vi "Response Type.vi"(8 "error in (no error)":errorcluster, 11 "http-client in":refnum<class "http-client.lvclass">) -> (0 "error out":errorcluster, 2 "response type":refnum<class "response.lvclass">, 3 "http-client out":refnum<class "http-client.lvclass">)   [LabVIEW 2020, in "http.lvlib" / "http-client.lvclass"]
uses:
  http-client.lvclass
  response/response.lvclass
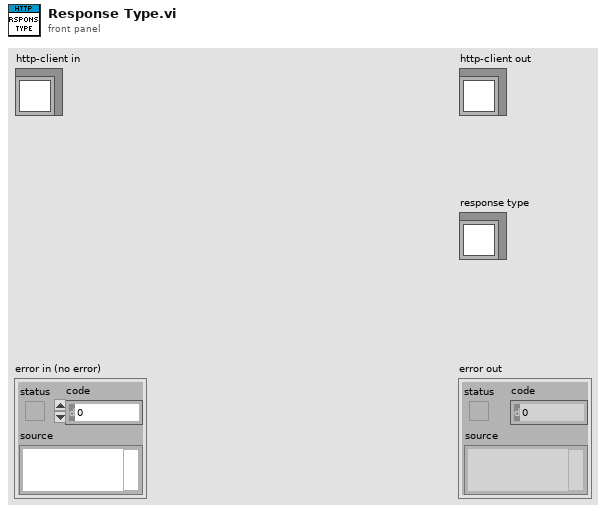
[diagram p1: front panel]
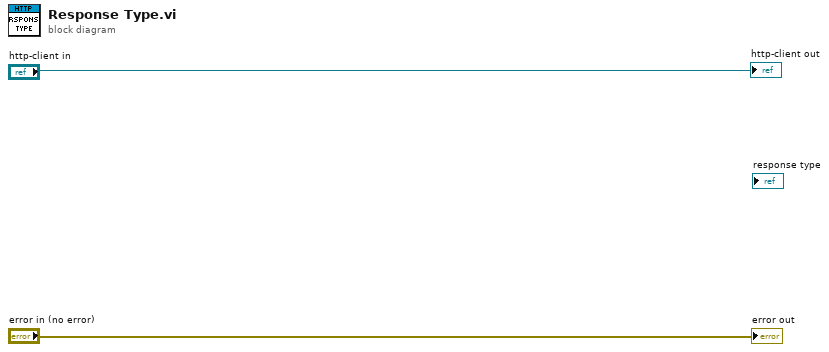
[diagram p0: block diagram]
diagram:
  "error out" <- "error in (no error)"
  "http-client out" <- "http-client in"
